vi "dfd_Sort Zeros for Minimum Phase.vi"(8 "tol":dbl=0.001, 10 "zeros":cdb[](array[numeric])) -> (0 "error":i32, 1 "zeros  in h0":cdb[](array[numeric]), 2 "zeros  in g0":cdb[](array[numeric]))   [LabVIEW 2017, in "NI_DigFilter_Design.lvlib"]
uses:
  <vilib>/addons/Digital Filter Design/NI_DigFilter_Design.lvlib
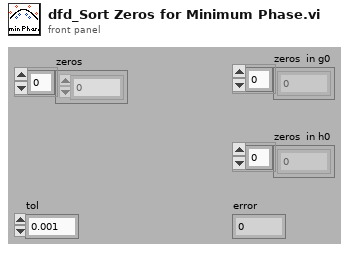
[diagram p1: front panel]
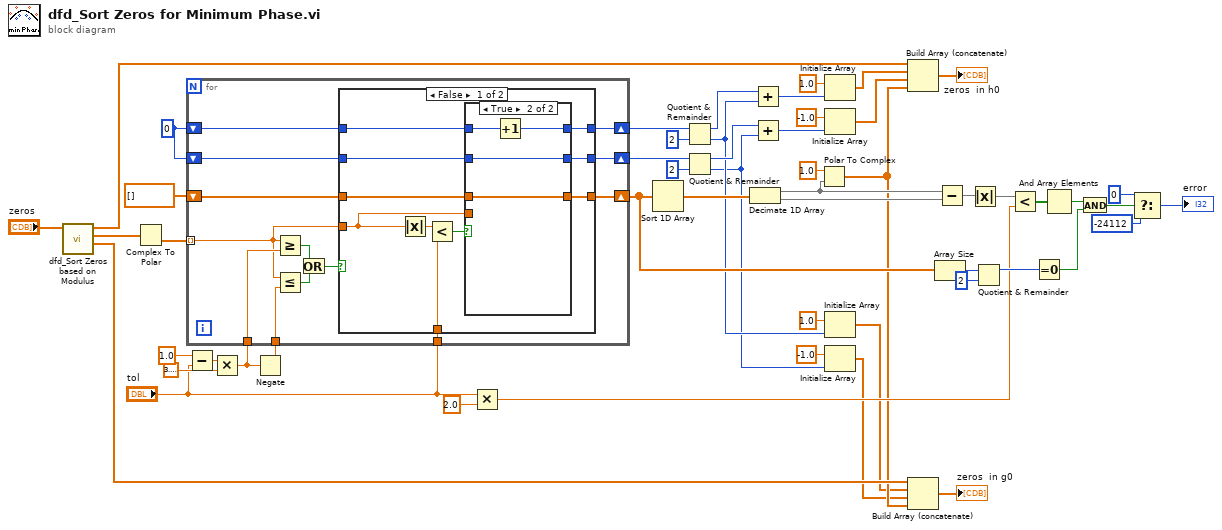
[diagram p0: block diagram]
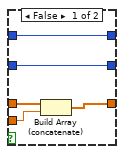
[diagram p2: hidden frame]
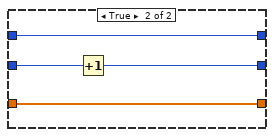
[diagram p3: hidden frame]
diagram:
  w41 = 0
  n1 = call <vilib>:"dfd_Sort Zeros based on Modulus.vi"("zeros"="zeros") -> (">1"=w20:cdb[], "=1"=w46:cdb[], "<1"=w49:cdb[])  [unwired: 8 out]
  n2 = Complex To Polar(r * e^(i*theta)=w46) -> (theta=w45:dbl[])  [unwired: 1 out]
  n3 = Subtract(x=1.0, y="tol") -> (x-y=w43:dbl)
  n4 = Multiply(x=w43, y=3.141592653589793) -> (x*y=w2:dbl)
  n5 = Negate(x=w2) -> (-x=w1:dbl)
  n6 = for {
    tunnel: w45 -> [w58] mode=indexing
    tunnel: w2 -> [w66]
    shift-right: [w61] -> w23
    shift-left: w41 -> [w62]
    shift-right: [w59] -> w21
    shift-left: w41 -> [w60]
    tunnel: "tol" -> [w57]
    shift-right: [w56] -> w39
    shift-left: dbl[] [] -> [w55]
    tunnel: w1 -> [w54]
    n7 = Greater Or Equal?(x=w58, y=w66) -> (x >= y?=w64:bool)
    n8 = Less Or Equal?(x=w58, y=w54) -> (x <= y?=w65:bool)
    n9 = Or(x=w64, y=w65) -> (x .or. y?=w63:bool)
    n10 = case shown="False" w63 {
      tunnel: w62 -> [w73 w88]
      tunnel: [w71 w88] -> w61
      tunnel: w60 -> [w72 w87]
      tunnel: [w70 w86] -> w59
      tunnel: w58 -> [w67 _]
      tunnel: w57 -> [w75 _]
      tunnel: [w68 w89] -> w56
      tunnel: w55 -> [w69 w89]
      frame False {
        n11 = Absolute Value(x=w67) -> (abs(x)=w76:dbl)
        n12 = Less?(x=w76, y=w75) -> (x < y?=w74:bool)
        n13 = case shown="True" w74 {
          tunnel: w73 -> [w81 w83]
          tunnel: w72 -> [w80 w84]
          tunnel: [w81 w82] -> w71
          tunnel: [w80 w84] -> w70
          tunnel: w69 -> [w79 w85]
          tunnel: w67 -> [w78 _]
          tunnel: [w77 w85] -> w68
          frame False {
            n14 = Build Array (concatenate)(w79, w78) -> (w77:dbl[])
          }
          frame True {
            n15 = Increment(x=w83) -> (x+1=w82:i32)
          }
        }
      }
      frame True {
        n16 = Increment(x=w87) -> (x+1=w86:i32)
      }
    }
  }
  n17 = Multiply(x="tol", y=2.0) -> (x*y=w29:dbl)
  n18 = Sort 1D Array(array=w39) -> (sorted array=w38:dbl[])
  n19 = Quotient & Remainder(x=w23, y=2) -> (x-y*floor(x/y)=w13:i32, floor(x/y)=w4:i32)
  n20 = Quotient & Remainder(x=w21, y=2) -> (x-y*floor(x/y)=w10:i32, floor(x/y)=w3:i32)
  n21 = Decimate 1D Array(w38) -> (w19:dbl[], w34:dbl[])
  n22 = Add(x=w13, y=w4) -> (x+y=w12:i32)
  n23 = Add(x=w10, y=w3) -> (x+y=w11:i32)
  n24 = Polar To Complex(1:w19, 2:1.0) -> (0:w7:cdb[])
  n25 = Initialize Array(1.0 ("element"), w12) -> (w15:dbl[])
  n26 = Initialize Array(-1.0 ("element"), w11) -> (w14:dbl[])
  n27 = Initialize Array(1.0 ("element"), w4) -> (w6:dbl[])
  n28 = Initialize Array(-1.0 ("element"), w3) -> (w5:dbl[])
  n29 = Build Array (concatenate)(w49, w15, w14, w7) -> (→"zeros  in h0":cdb[])
  n30 = Build Array (concatenate)(w20, w6, w5, w7) -> (→"zeros  in g0":cdb[])
  n31 = Array Size(array=w39) -> (size(s)=w37:i32)
  n32 = Subtract(x=w19, y=w34) -> (x-y=w33:dbl[])
  n33 = Absolute Value(x=w33) -> (abs(x)=w32:dbl[])
  n34 = Quotient & Remainder(x=w37, y=2) -> (x-y*floor(x/y)=w35:i32)  [unwired: 1 out]
  n35 = Less?(x=w32, y=w29) -> (x < y?=w28:bool[])
  n36 = Equal To 0?(x=w35) -> (x = 0?=w26:bool)
  n37 = And Array Elements(Boolean array=w28) -> (logical AND=w27:bool)
  n38 = And(x=w27, y=w26) -> (x .and. y?=w25:bool)
  n39 = Select(t=0, s=w25, f=-24112) -> (s? t:f=→"error":i32)
